vi "manipulation des tableaux.vi"() -> ()   [LabVIEW 2014]
panel:
  in  "supprimer":bool
  in  "numero d'element a suprimer":i32
  in  "element a inserer":dbl
  in  "index":i32
  in  "inserer":bool
  in  "trie":bool
  in  "initialisation":bool
  out "nbr lement":i32
  out "Multiplication":dbl
  out "somme":dbl
  in  "Array":dbl[](array[numeric])
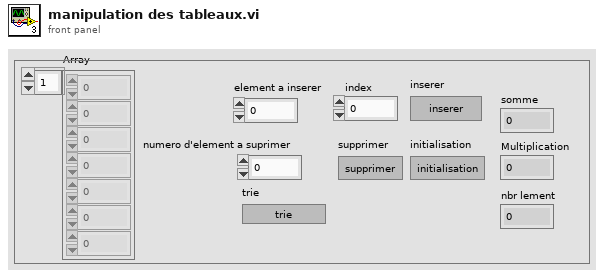
[diagram p1: front panel]
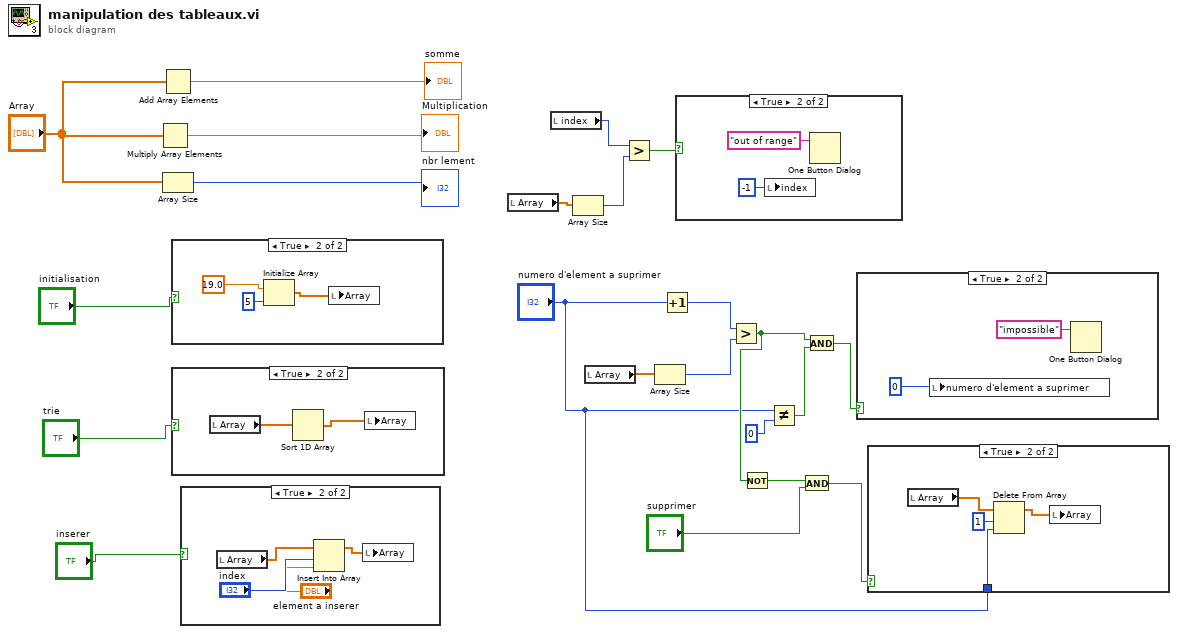
[diagram p0: block diagram]
diagram:
  n1 = Multiply Array Elements(1:"Array") -> (0:→"Multiplication":dbl)
  n2 = Add Array Elements(numeric array="Array") -> (sum=→"somme":dbl)
  n3 = Array Size(array="Array") -> (size(s)=→"nbr lement":i32)
  n4 = case shown="True" "initialisation" {
    frame False {
    }
    frame True {
      n5 = Initialize Array(19.0, 5 ("dimension size")) -> (w23:dbl[])
      n6 = local write "Array"(w23) -> ()
    }
  }
  n7 = case shown="True" "trie" {
    frame False {
    }
    frame True {
      n8 = local read "Array"() -> (w27:dbl[])
      n9 = Sort 1D Array(array=w27) -> (sorted array=w26:dbl[])
      n10 = local write "Array"(w26) -> ()
    }
  }
  n11 = case shown="True" "inserer" {
    frame False {
    }
    frame True {
      n12 = local read "Array"() -> (w31:dbl[])
      n13 = Insert Into Array(array=w31, index="index", new element="element a inserer") -> (w30:dbl[])
      n14 = local write "Array"(w30) -> ()
    }
  }
  n15 = local read "Array"() -> (w14:dbl[])
  n16 = local read "index"() -> (w15:i32)
  n17 = Array Size(array=w14) -> (size(s)=w13:i32)
  n18 = local read "Array"() -> (w10:dbl[])
  n19 = Greater?(x=w15, y=w13) -> (0:w12:bool)
  n20 = Array Size(array=w10) -> (size(s)=w9:i32)
  n21 = Increment(x="numero d'element a suprimer") -> (x+1=w11:i32)
  n22 = case shown="True" w12 {
    frame False {
    }
    frame True {
      n23 = local write "index"(-1 ("index")) -> ()
      n24 = One Button Dialog(message="out of range") -> ()  [unwired: 1 in, 1 out]
    }
  }
  n25 = Greater?(x=w11, y=w9) -> (0:w5:bool)
  n26 = Not(x=w5) -> (.not. x?=w4:bool)
  n27 = Not Equal?(x="numero d'element a suprimer", y=0) -> (x != y?=w8:bool)
  n28 = And(x=w4, y="supprimer") -> (x .and. y?=w2:bool)
  n29 = And(x=w5, y=w8) -> (x .and. y?=w7:bool)
  n30 = case shown="True" w7 {
    frame False {
    }
    frame True {
      n31 = local write "numero d'element a suprimer"(0) -> ()
      n32 = One Button Dialog(message="impossible") -> ()  [unwired: 1 in, 1 out]
    }
  }
  n33 = case shown="True" w2 {
    tunnel: "numero d'element a suprimer" -> [_ w37]
    frame False {
    }
    frame True {
      n34 = local read "Array"() -> (w39:dbl[])
      n35 = Delete From Array(array=w39, length=1, index=w37) -> (array with subset deleted=w36:dbl[])  [unwired: 1 out]
      n36 = local write "Array"(w36) -> ()
    }
  }
